vi "Get Image Names in Directory.vi"(8 "error in (no error)":errorcluster, 10 "Image Path":string, 11 "CCDCamera in":refnum<class "CCDCamera.lvclass">) -> (0 "error out":errorcluster, 3 "CCDCamera out":refnum<class "CCDCamera.lvclass">)   [LabVIEW 2018, in "CCDCamera.lvclass"]
uses:
  CCDCamera.lvclass
  Interface/Interface.lvclass
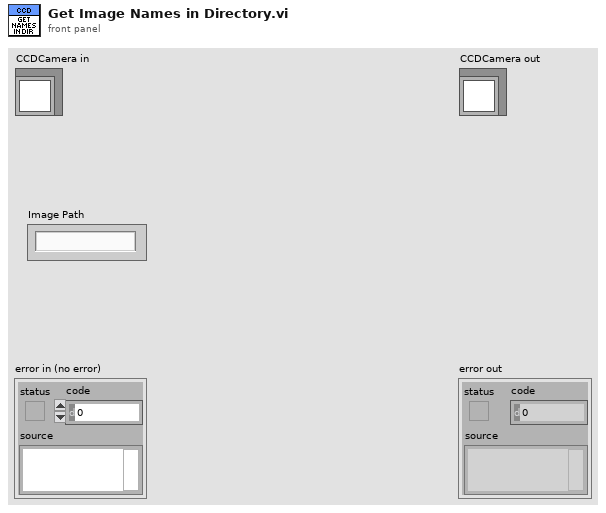
[diagram p1: front panel]
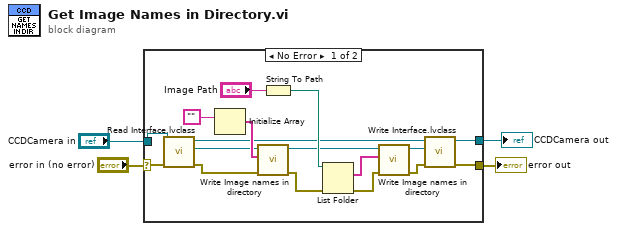
[diagram p0: block diagram]
diagram:
  n1 = case shown="No Error" "error in (no error)" {
    selector: "error in (no error)" -> [w18 w23]
    tunnel: [w15 w23] -> w3
    tunnel: [w16 w22] -> w1
    tunnel: "CCDCamera in" -> [w17 w22]
    frame No Error {
      n2 = call-dynamic "Read Interface.lvclass.vi"("error in (no error)"=w18, "CCDCamera in"=w17) -> ("error out"=w12:errorcluster, "Interface.lvclass"=w13:refnum<class "Interface.lvclass">, "CCDCamera out"=w5:refnum<class "CCDCamera.lvclass">)  [unwired: 7 in]
      n3 = Initialize Array("") -> (w14:string[])  [unwired: 1 in]
      n4 = call "Write Image names in directory.vi"("error in (no error)"=w12, "Image names in directory"=w14, "Interface in"=w13) -> ("error out"=w11:errorcluster, "Interface out"=w8:refnum<class "Interface.lvclass">)  [unwired: 7 in]
      n5 = String To Path(string="Image Path") -> (path=w20:path)
      n6 = List Folder(path=w20, error in=w11) -> (filenames=w9:string[], error out=w10:errorcluster)  [unwired: 2 in, 2 out]
      n7 = call "Write Image names in directory.vi"("error in (no error)"=w10, "Image names in directory"=w9, "Interface in"=w8) -> ("error out"=w7:errorcluster, "Interface out"=w6:refnum<class "Interface.lvclass">)  [unwired: 7 in]
      n8 = call-dynamic "Write Interface.lvclass.vi"("error in (no error)"=w7, "Interface.lvclass"=w6, "CCDCamera in"=w5) -> ("error out"=w15:errorcluster, "CCDCamera out"=w16:refnum<class "CCDCamera.lvclass">)  [unwired: 7 in]
    }
    frame Error {
    }
  }
  "error out" <- w3
  "CCDCamera out" <- w1
